vi "theta2enc.vi"(9 "th 2":dbl, 10 "th 1":dbl) -> (1 "enc 2":i32, 2 "enc 1":i32)   [LabVIEW 2018]
uses:
  <vilib>/imath/engines/lvmath2/RunTimeEngine/BuiltInFunctions/int32/NIMS_int32(real).vi
  <instcachedir>/0/NIMS_int32(real)_9F6AE75EF4BE45429513317A1C5A7040.lvgen/NIMS_int32(real)_9F6AE75EF4BE45429513317A1C5A7040_000.vi
  <vilib>/imath/engines/lvmath2/RunTimeEngine/NodeEndStatement/NIMS_NodeEndStatement_Output.vi
  <instcachedir>/0/NIMS_NodeEndStatement_Output_53EC0D466D134D7ABD903AC30B43404B.lvgen/NIMS_NodeEndStatement_Output_53EC0D466D134D7ABD903AC30B43404B_011.vi
  <vilib>/imath/engines/lvmath2/RunTimeEngine/ErrorHandling/NIMS_Finalize Error.vi
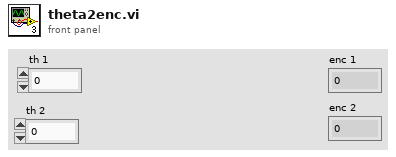
[diagram p1: front panel]
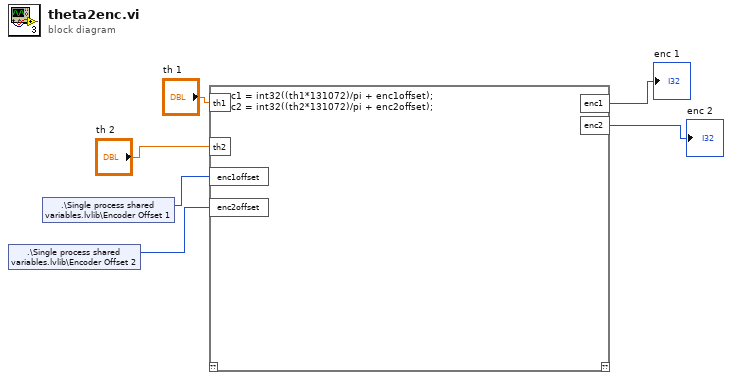
[diagram p0: block diagram]
diagram:
  n1 = shared-variable ".\\Single process shared variables.lvlib\\Encoder Offset 2"() -> (w1:i32)  [unwired: 1 in, 1 out]
  n2 = shared-variable ".\\Single process shared variables.lvlib\\Encoder Offset 1"() -> (w2:i32)  [unwired: 1 in, 1 out]
  n3 = mathscript code="enc1 = int32((th1*131072)/pi + enc1offset);\nenc2 = int32((th2*131072)/pi + enc2offset);"("th1"="th 1", "th2"="th 2", "enc1offset"=w2, "enc2offset"=w1) -> ("enc1"=→"enc 1":i32, "enc2"=→"enc 2":i32)  [unwired: 1 in, 1 out]
